vi "VDI Write Bytes.vi"(1 "AftClkCnt":u16, 4 "PreClkCnt":u16, 5 "WriteLen":u8, 6 "pWriteData":u8[](array[numeric]), 7 "Addr":u8, 9 "Channel":u8, 10 "DevIndex":i32, 11 "DevType":i32) -> (2 "function return":i32, 3 "pWriteData out":u8[](array[numeric]))   [LabVIEW 2010, in "ControlDigRF.lvlib"]
doc: "int WINAPI VDI_WriteBytes(int DevType,int DevIndex,unsigned char Channel,unsigned char Addr,unsigned char *pWriteData,unsigned char WriteLen,unsigned short PreClkCnt,unsigned short AftClkCnt);"
uses:
  ControlDigRF.lvlib
  ControlDigRF/Ginkgo_Driver.dll
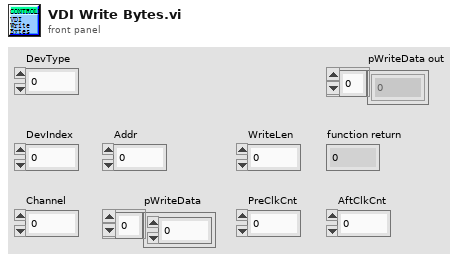
[diagram p1: front panel]
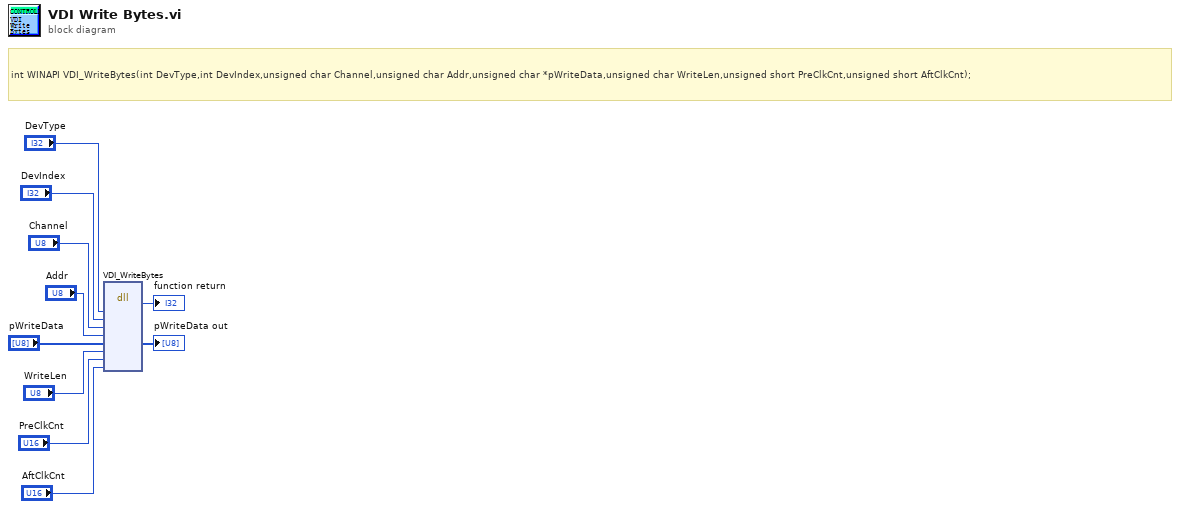
[diagram p0: block diagram]
diagram:
  # "int WINAPI VDI_WriteBytes(int DevType,int DevIndex,unsigned char Channel,unsigned char Addr,unsigned char *pWriteData,unsigned char WriteLen,unsigned short PreClkCnt,unsigned short AftClkCnt);"
  n1 = dll-call lib="E:/Project/vt_ginkgo/truck/Ginkgo Driver/vs2010/Ginkgo_USB-I2C&SPI&CAN_API_v2.0.3.3/lib/labview_32bit/ControlDigRF/Ginkgo_Driver.*" fn="VDI_WriteBytes"("DevType"="DevType", "DevIndex"="DevIndex", "Channel"="Channel", "Addr"="Addr", "pWriteData"="pWriteData", "WriteLen"="WriteLen", "PreClkCnt"="PreClkCnt", "AftClkCnt"="AftClkCnt") -> (→"function return":i32, "pWriteData"=→"pWriteData out":u8[])  [unwired: 10 in, 2 out]
